vi "Initialize Neopixel.vi"(10 "Digital Output":refnum<k21>, 11 "Neopixel FIFO":T1="Neopixel FIFO") -> (3 "Neopixel - FPGA Out":refnum<class "Neopixel - FPGA.lvclass">)   [LabVIEW 2021, in "Neopixel - FPGA.lvclass"]
uses:
  Neopixel - FPGA.lvclass
  Controls/Neopixel FIFO.ctl
  Controls/FPGA Resources.ctl
  Neopixel - FPGA.lvclass/Neopixel - FPGA.ctl
  Private/Controls/Raw Frame Memory.ctl
  <vilib>/rvi/LocalResourceManager/LocalResourceManager.xnode
  <vilib>/rvi/DataTransferAndStorage/Container/Common/niFpgaContainerGetUniqueNameForEmu.vi
  <vilib>/rvi/DataTransferAndStorage/Container/Common/niFpgaContainerSetEmuInfo.vi
  <vilib>/rvi/eio/common/nirviEmuReportErrorAndStop.vi
  Private/Controls/Number Of Neopixels.ctl
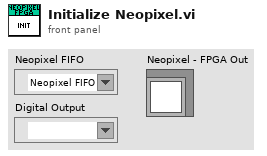
[diagram p1: front panel]
types:
  T1 = typedef "Neopixel - FPGA.lvclass/Neopixel FIFO.ctl" = refnum<k21>
  T2 = typedef "Neopixel - FPGA.lvclass/FPGA Resources.ctl" = cluster{"Neopixel FIFO":T1, "Digital Output":refnum<k21>, "Raw Frame Memory":T3, "Number of Neopixels Register":T4}
  T3 = typedef "Neopixel - FPGA.lvclass/Raw Frame Memory.ctl" = refnum<k21>
  T4 = typedef "Neopixel - FPGA.lvclass/Number Of Neopixels.ctl" = refnum<k21>
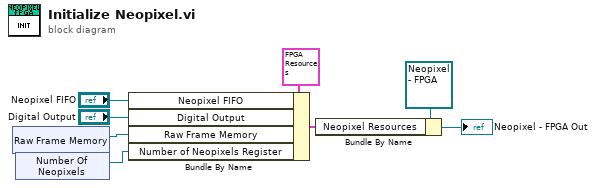
[diagram p0: block diagram]
diagram:
  n1 = xnode "Raw Frame Memory"() -> ("Memory Out"=w1:refnum<k21>)
  n2 = xnode "Number Of Neopixels"() -> ("Register Out"=w2:refnum<k21>)
  n3 = Bundle By Name(cluster=T2 {"Neopixel FIFO"="Neopixel FIFO", "Digital Output"="ConnectorC/DIO0", "Raw Frame Memory"="Raw Frame", "Number of Neopixels Register"="Register"} ("Neopixel Resources"), "Neopixel FIFO"="Neopixel FIFO", "Digital Output"="Digital Output", "Raw Frame Memory"=w1, "Number of Neopixels Register"=w2) -> (w4:T2)
  n4 = Bundle By Name(cluster=refnum<class "Neopixel - FPGA.lvclass"> refnum ("Neopixel - FPGA Out"), "Neopixel Resources"=w4) -> (→"Neopixel - FPGA Out":refnum<class "Neopixel - FPGA.lvclass">)
